vi "To Byte Array (EEPROM Device Data Header).vi"(1 "Device Data Header":T1={"Checksum"=0, "Number of Channels"=0, "Number of Attenuations"=[], "Number of Attenuator Settings"=[], "Number of Gain Settings"=[], "Pointer to Cal Data"=[], "Number of Reserved Bytes"=7, "Number of Frequencies"=[]} {"Checksum" format="%x"}) -> (0 "byte array out":u8[](array[numeric]) format="%x")   [LabVIEW 2013]
uses:
  <instrlib>/ni579x/Config/v1/Shared/Types/EEPROM/ni579x EEPROM Device Data Header.ctl
  <instrlib>/ni579x/Config/v1/Shared/Conversions/To Byte Array (U8).vi
  <instrlib>/ni579x/Config/v1/Shared/Conversions/To Byte Array (U32).vi
  <instrlib>/ni579x/Config/v1/Shared/Conversions/To Byte Array (U16).vi
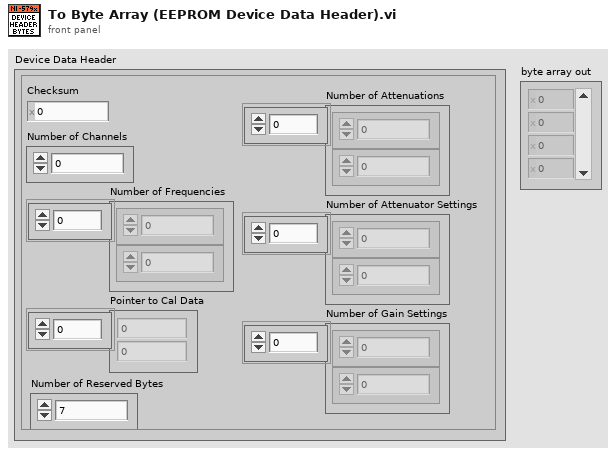
[diagram p1: front panel]
types:
  T1 = typedef "ni579x EEPROM Device Data Header.ctl" = cluster{"Checksum":u32, "Number of Channels":u8, "Number of Attenuations":u16[], "Number of Attenuator Settings":u8[], "Number of Gain Settings":u8[], "Pointer to Cal Data":u32[], "Number of Reserved Bytes":i32, "Number of Frequencies":u16[]}
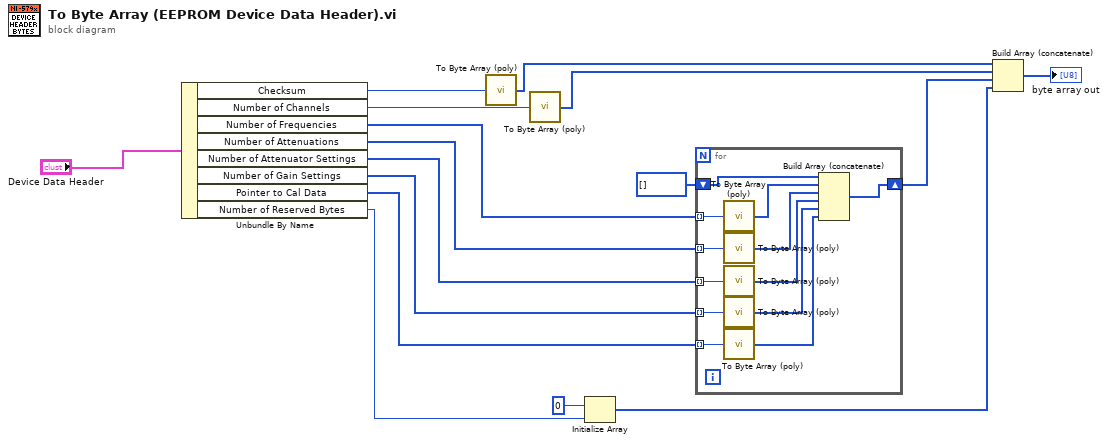
[diagram p0: block diagram]
diagram:
  n1 = Unbundle By Name("Device Data Header") -> ("Checksum"=w16:u32, "Number of Channels"=w15:u8, "Number of Frequencies"=w3:u16[], "Number of Attenuations"=w14:u16[], "Number of Attenuator Settings"=w13:u8[], "Number of Gain Settings"=w12:u8[], "Pointer to Cal Data"=w11:u32[], "Number of Reserved Bytes"=w8:i32)
  n2 = call-poly <instrlib>:"To Byte Array (poly).vi"("element in"=w16) -> ("byte array out"=w7:u8[])
  n3 = call-poly <instrlib>:"To Byte Array (poly).vi"("element in"=w15) -> ("byte array out"=w6:u8[])
  n4 = Initialize Array(u8 0, w8) -> (w1:u8[])
  n5 = for {
    tunnel: w14 -> [w28] mode=indexing
    tunnel: w13 -> [w27] mode=indexing
    tunnel: w12 -> [w26] mode=indexing
    tunnel: w11 -> [w25] mode=indexing
    shift-right: [w20] -> w2
    shift-left: u8[] [] -> [w18]
    tunnel: w3 -> [w19] mode=indexing
    n6 = call-poly <instrlib>:"To Byte Array (poly).vi"("element in"=w19) -> ("byte array out"=w17:u8[])
    n7 = call-poly <instrlib>:"To Byte Array (poly).vi"("element in"=w28) -> ("byte array out"=w24:u8[])
    n8 = call-poly <instrlib>:"To Byte Array (poly).vi"("element in"=w27) -> ("byte array out"=w23:u8[])
    n9 = call-poly <instrlib>:"To Byte Array (poly).vi"("element in"=w26) -> ("byte array out"=w22:u8[])
    n10 = call-poly <instrlib>:"To Byte Array (poly).vi"("element in"=w25) -> ("byte array out"=w21:u8[])
    n11 = Build Array (concatenate)(w18, w17, w24, w23, w22, w21) -> (w20:u8[])
  }
  n12 = Build Array (concatenate)(w7, w6, w2, w1) -> (→"byte array out":u8[])
